vi "Principal Component Regression vs Partial Least Squares Regression.vi"() -> ()   [LabVIEW 2020]
doc: "Created a simple data set with two features. Fitting a PCA estimator to display the two principal components of this data set, i.e., the two directions that explain the most variance in the data."
uses:
  Model/Unsupervised/Decomposition/PCA/Controls/pca_params.ctl
  Model/Unsupervised/Decomposition/PCA/PCA.lvclass
  C:/Users/cipop/TDF Dropbox/2_Technologies de France/1 - Services et Etudes/PLAIY/2 - DEV/PLAIYLAB/code/Model/Model.lvclass
  Model/Unsupervised/Decomposition/PCA/PCA.vi
panel:
  in  "error in":errorcluster
  in  "X":dbl[][](array[numeric])=[[-3.1230621555120366, -3.267402245779568], [-2.7759583555493745, -0.9291009956420317], [-2.5824162791620315, -4.072344785760595], [-1.4924533321482034, -1.9203606695549433], [-0.04152867510525987, 0.38116552193039455], [-0.9895929568838566, 0.35548272004878073], [-1.321002512421451, -1.4319109557167145], [-0.9062030407418514, -0.7201426317829231], [-2.363965378211708, -3.00551409310223], [-0.07622116200586487, -0.9848213835175939], [3.8827997801273813, 5.2682947183614415], [-1.0455682933772348, -2.0118262855175173], [-3.000793770679625, -5.066072884305923], [0.021076191053119836, -0.1712349292866861], [-3.293213004454131, -2.348044580088958], [-0.45156251453811036, -0.13684672563754458], [2.4911990537849347, 0.8654600606814207], [0.49437031989305863, 0.7473930976389208], [-2.6551906571871515, -1.8746011462978966], [0.7965278046955226, 0.6235436957786513], [2.4672057894742827, 1.4246706773928945], [1.8127458791245286, 4.183723187879213], [1.0689101490798731, 0.8028309544259182], [1.6693409342820642, 2.7851759352048475], [2.7779867409191974, 3.056413113478895], [1.28044097132362, 1.9168718091876966], [1.454516472193804, 0.4800380543766737], [-0.17474077869416443, 0.2424933474987974], [-0.2662603373981937, 0.002593279598261611], [1.2360847889518942, 1.079101339057454], [1.2974868876792334, 1.1549241930603973], [2.236292462300943, 0.8312098407203671], [-0.08570535170975882, -0.5221219961580871], [2.4558730848103254, 3.383922938130942], [1.473082668462659, 1.793339539503028], [-1.2719644066222633, -1.366366853019776], [-1.2455615883649316, -2.764076488877849], [-0.31128133394330143, -1.084938213482685], [1.7386890479593449, 1.4459865694538756], [0.4860291194557282, 0.6325831741811381], [1.4607162202673052, 2.668123312217531], [0.023997601243387456, -1.581210861785806], [-3.4400020907207445, -2.0744427796423204], [-1.8557584770801652, -2.3791586256349135], [1.2252785308669916, 2.5511532590490686], [0.03485131421930365, 1.3219094827980622], [-0.8489718087252514, 0.021057633347454585], [-0.954242520882054, -0.3861611991001935], [-0.9401672768593397, 0.7612455190095062], [-0.41752715405613133, -0.07170568835595528], [-2.4167558580489956, -4.2649463448703555], [1.5994216853420016, 2.903701384378012], [0.935056942906058, 3.140150593548995], [1.0700158249093736, 0.4799948638084063], [-3.943985606858868, -3.1045675966732573], [-3.555582951142261, -3.2479521887428753], [0.436774411909285, 2.516790560089131], [0.028405354509702996, 0.8742736180556507], [-1.4858766331534665, -1.9164243034844521], [-1.4917113621038822, -0.7947003467271441], [-0.054206900478580566, -1.2158431671974066], [-1.178420764227316, -0.0014102617409005314], [1.2255635582681221, 1.2899555529512825], [-0.23618032716024984, 1.658692026165808], [-1.3219687145720118, -1.133629585524625], [0.9941620940232232, 1.7385461989049822], [1.0983431465659563, 1.329899833217794], [0.7016338957803231, 1.5369575037307723], [-0.8455726116795177, -1.2164018547360114], [-0.08985373180301681, -1.251281106760939], [2.2382660497620366, 3.102539909775831], [-0.6036790814168229, -0.04728997705352106], [-4.427797625785037, -4.237298506790273], [0.9318628713293798, 2.27033725141622], [2.4139407399635457, 2.365954334709854], [-0.7725163598260496, 0.8831626619431198], [1.6582548882395716, 1.0916356936402005], [0.5055970555135226, -0.09829604362883215], [-1.304497377056593, -2.671363413465319], [2.123201941989344, 2.0476470765576895], [-0.1737072849012109, 1.8165369702193837], [-1.6148002860594206, -1.8144794467292016], [1.5895553483051157, 2.7610553746046356], [2.4517586006380316, 1.2757306514269526], [-2.127795936579116, -2.1797146955158735], [-1.687037561069112, -1.657546670957851], [-1.0800891896009337, -1.95708907640884], [1.357587098949138, 2.3166917679275847], [1.684487467372001, 1.2660220463726513], [0.744043644169997, 0.8966271774157081], [1.295689925648856, 0.0889593754981145], [2.212908959730294, 0.28276797927442476], [-0.20579022578061912, -1.921420302525838], [1.798785393093465, 2.178048879910527], [0.4253096343310593, 2.118694225099275], [1.9993280061041725, 2.6399196575033486], [0.6685277864008033, -0.4346535641530578], [-0.776425902433697, -1.0962709897646585], [-1.7014334411694816, -1.1456806529369103], [-4.266831862548306, -3.6365313912391892], [0.7340165938152251, 0.6156773915555652], [-2.156524327626228, -1.8591647387793435], [-0.22272426785381416, -1.9570194715144735], [0.42157644704371794, -0.2755886336250671], [-0.412047724827981, -0.5892392529116066], [-1.6686018074550817, -1.637365447685474], [-1.0589271731939833, -1.7386939359527704], [1.7732203834350928, 1.6636029951994373], [-0.16778048582484578, 0.19918313987653768], [-3.713200926998545, -4.4275600057892115], [1.7591241647054534, 1.714087615107567], [0.5176111003363346, 1.1154727511926705], [2.5145201228572627, 3.034571758319521], [-0.37870731488022336, -0.20379042066372643], [1.110409630266099, 1.0615214579176058], [2.609136057527492, 2.5631252879627286], [0.6824611972822181, 1.2415185537957432], [1.5077068204105204, 2.59825790632907], [-1.4010279076116303, -3.8226036325343458], [-1.0544580831604022, -0.5355421839959715], [1.259077266138524, 1.0700649156531268], [0.37355186176683475, 0.1289644719074876], [1.3768906865528834, -0.1306023050172932], [-2.462876330674744, -1.7761999881369224], [2.1023768285563813, 0.9453840523307628], [-0.5638865499045511, -1.2689050210099266], [-0.06966776486358095, -0.41680386605849484], [-1.502231764160231, -1.045428970358411], [1.9143630858651652, 0.8104645184180699], [2.301476515109009, 3.356302996730963], [2.2272802260543494, 2.0982191939319432], [1.0129753127016978, 1.1407019415196935], [3.1034650485695434, 3.861303032071852], [-0.9117744561650152, -0.9836728847040506], [0.463620329133252, 0.6493326540176726], [0.7729816660272796, -1.9924010730560782], [-3.4350402393224906, -3.646224067737516], [1.2805629784436563, 1.102047845501593], [-0.7562481528851783, -1.0143643627180428], [2.2902989516589423, 4.866598705110763], [-0.34440836486571075, 0.6622855101700247], [0.35019181744509975, 2.023066391831823], [-0.7879831666210565, -0.29229068871313707], [1.102155845873062, 2.5699813382136005], [-1.8130912584448788, -0.7763241349282213], [1.2868996412809248, 1.0151567928103926], [-3.2610412289082293, -4.960120115268076], [-0.3627145013656148, 0.7629632300366], [-0.4627849749446247, 0.06446751141708973], [0.4691415755908187, 0.9415146073433274], [1.3031172548670646, 3.2755197421109115], [0.5468129888226406, -0.06713894944707846], [-0.8635821125135921, -1.5021255953649117], [2.9016510378335933, 2.014313751071669], [-1.0644734160420157, -1.4237555499359422], [-0.3358678897271853, 0.7326850594809373], [2.240403391217416, 1.8791685691338935], [0.5875201531303886, 0.7923974655491977], [0.21795943160435005, -0.04328232332688953], [0.15732693404684453, 0.07329332353105325], [1.6097290944355735, 1.048439962492894], [0.006536589845641649, -0.9257051563936818], [2.074682549867369, 2.1218886778081125], [-0.9054603158856454, 1.2955334831430163], [0.6775848894798995, 1.7881265800876855], [-0.6208732812742819, -1.9785867891528066], [-0.6665796080587857, -2.027235361483064], [4.082778804652155, 5.454806295039896], [2.6697866153395244, 3.6240263333178833], [0.27325472064938794, 2.0612956521081696], [-1.5321575468236415, -2.2836685408424118], [1.7644644634471083, 0.8108784741798338], [0.8737903876842514, 0.7377434932758122], [0.5219295476248138, 0.7802974932957978], [-1.1370742912796614, -0.9759344513891441], [2.0062115379467023, 0.8618636827982649], [-1.8995543846428702, -2.964692117125013], [1.3476694183914666, 1.0448147458438994], [3.2939016371559027, 3.387541996156069], [0.4723993359108689, 1.2076047997409527], [-1.15662143970013, -1.3613950313055445], [-1.716179145733433, -1.669696577670932], [-0.05723075688290312, 0.10104753431650992], [0.5192135789425586, 0.19922298559988247], [1.0254855678930572, 0.02871548705687116], [0.04955493009300638, -0.9820086854769112], [-1.2624628154709912, -1.751647832684781], [-0.33700311796421617, 0.11957927435606289], [-0.25192758744399957, -1.9429496323234021], [-0.11276460560748963, 0.7890587860400128], [2.6071499866693078, 3.4833953040787584], [4.257203373914415, 3.954168641112636], [0.7922075925398219, -0.8005885735062946], [2.3897611827611946, 1.2789610808487466], [-2.8095189142448405, -3.1444626915200535], [-0.8227685231847532, -1.2045447824707207], [1.4195621605189146, -0.017860496326389086], [0.8759428355501255, 0.23619224516754922], [-2.0079386658467873, -1.1747473904713763], [-2.865050676141875, -2.4888510666693113], [1.5662955642224357, 0.6798126138498647], [-1.451535919349128, -1.3401888755973128], [2.7400188171811104, 3.606925876978513], [-1.376993484663037, -1.5637493342400972], [0.7232607799336566, 0.007598693396809408], [1.9778409324743031, 3.173243734894971], [0.6316594322042454, 0.5010434202148424], [-3.2181946114229407, -3.081792175376673], [-0.6864464432967216, -0.6614831723449329], [-3.4013792813625985, -2.213561355763916], [-1.8374875875250434, -1.5590783880981642], [3.3988179387222597, 4.141794841306994], [0.16654151049915855, 0.29503147353814235], [-0.14335429990191018, -3.0396133959544915], [0.8017062074067494, 1.2291641515886955], [1.5039328123750066, 0.29082534424293593], [-1.5796173846581025, -1.5745941219067074], [1.442732420989098, 2.032925902941954], [-1.3609610156158853, -1.6010154518183417], [-1.3639140932992975, -1.5280525761180117], [1.2524880357581751, 0.263775174168296], [0.04166216316219769, 0.25274334155968015], [-1.3884268772571104, -1.7595823133499298], [-0.25774689097973547, -1.3148944148621475], [1.3508653136453304, 1.4789869785616112], [1.319642108393654, 2.4171677862715444], [-0.9098526917261823, -0.7816334494516979], [-1.6045976678183593, 0.22330509901165885], [1.91266109902782, -0.04865305233923711], [-0.3033301385811629, -0.41108709899179996], [1.3613388751841846, 0.5814760612414922], [0.632355175149752, 0.936460484967083], [-0.41533709348972814, 2.037264740613474], [1.9977090040313212, 1.5272587977725598], [3.6535437912370616, 4.5763467787299845], [3.612227162303425, 3.6988987613221695], [0.8224681920434698, 0.22730150377680097], [-3.3884945786544756, -2.958146009832311], [-1.7247957159551681, -2.96057279232882], [-2.122062605534064, -1.985345376811369], [-1.8072097919734924, -1.0547854685641302], [1.7216027059795702, 1.5877217080760038], [-0.05379126994125172, -2.845819232819154], [-2.7876170627020302, -2.711149183584468], [-0.038385718854680465, 0.1857154274986857], [1.883490221475557, 1.8567462235195495], [-2.489688174081815, -1.5790267308510786], [-4.41913520359936, -5.294065876287195], [1.3544232356882078, 1.060074551262173], [1.7232325775049468, 1.9526385876044559], [-0.615030305926815, -0.7618949409584685], [-1.6914289859234148, -2.2420553953822284], [0.8747548071075235, 0.4236121756401645], [3.5091420955780626, 2.4998362030706187], [1.27687209844225, 2.8708172038884943], [-2.190505332938247, -1.1452401661616056], [3.2196240049641918, 1.7380893892952531], [1.0003390332616595, 1.3650680508415156], [-1.3659393450364132, -0.5144656038865167], [-1.3704498241145897, 0.20805110086691792], [0.8398198656834015, 0.03473116745726451], [3.2387065698138966, 2.8917800427617566], [0.058962729271365366, -0.8615186312394935], [-2.278389544426113, -1.2098377112514116], [3.470865465231734, 5.0024962258386205], [3.4949949933122344, 4.546358154349681], [-2.058440133756621, -2.361956666208289], [2.4180605806504833, 2.241062225498926], [0.5267170334118553, 0.4308287856899863], [0.3922037650228464, 0.3478556487629465], [0.2715833857303947, -0.9456422148243377], [-0.38442623363554035, 1.1368986505003955], [0.8652291962581795, 0.5563569598142126], [-0.4600485979263118, -3.224354540600303], [-1.626505068926789, -2.5820772426607976], [-0.3207747770394916, -0.27774500504463906], [-1.4197924698318296, -1.9563707196356495], [0.45026329081991656, 1.8912850277911297], [3.897889263120339, 4.622608344846892], [2.6218847009640864, 2.2971224664694376], [-3.301918503358635, -3.9445072182586447], [0.5980983822673835, -1.1605311515703456], [1.1036727988509758, 1.5087773664099555], [-0.9052394846508768, -0.4222806869356237], [-0.286581152326219, 0.21385028561419794], [0.19529611899377375, -1.6864994254797279], [-0.45797349218007305, 0.26392005357943715], [-0.787159479405164, -1.3104294108592958], [1.9097056113668347, 1.08266442595462], [-0.3688384402389152, 0.7517408306763018], [3.5676609796297547, 3.520106901625024], [1.4786852325384499, 2.567937854862507], [1.1595631764060415, 0.8757262854092012], [0.12850885753191696, 0.6183429331979667], [2.222714982741702, -0.567649868791737], [-1.1250561201613922, -0.8680941797234533], [0.9230918926925015, -0.0460834151304334], [-0.7775161318321409, -0.5204978618967042], [0.8890384675958839, 0.8224028249598483], [1.6299947777113484, 1.737034604623724], [2.347493068162403, 3.208352087278317], [1.4381732475048934, 1.9471698344513608], [2.6292039709584474, 2.485461468307296], [1.0407882049782182, -0.5113238220891487], [0.005556324020851849, -0.3906779705754937], [3.5538439803439412, 2.829750673293757], [-1.4631289312303253, -0.7888821295209305], [0.008916586803490834, 0.4345989941153663], [-0.5403782600839842, -0.29254559504645045], [-1.347250555438185, -3.1692744353522677], [-0.920914319924806, -1.4873378096284238], [0.5269204220638951, 0.3053384009313589], [1.2537940139225603, 0.19535523435154833], [-1.1665147265552531, 0.37364057244978105], [0.093513478034955, 0.1089378355044669], [1.1969289497510778, 1.2898479034071806], [-0.579340808299716, -1.0717958934999747], [0.5418401684343338, 1.0621254821343125], [1.3871518540368202, 1.9020213022562555], [-2.058859870450213, -1.0055698351979978], [-0.5572580743889034, 0.7750252777585079], [-1.1952913305741795, -2.454736836780727], [2.1710504585102037, 2.2433254470564026], [-1.663659229548592, -2.0396197532244917], [0.1909057669573675, 1.8516586246375306], [0.7248117751784309, -1.5757000392352194], [-0.7930419116869436, -0.39130242838598306], [-0.6053496502382718, -0.24342308533023335], [0.7924702194679163, -0.4458178435735871], [1.1014650790503557, 0.3095040631620988], [2.194647815974929, 1.2673645533636786], [-0.7986299734995203, -0.8401842278411138], [1.076427371070743, 0.590361557660835], [-0.5189273666607129, 0.5181107389127977], [3.1185796730324777, 4.07621747192674], [1.8759760425434933, 0.24001455309733133], [3.6882511189370213, 3.397501359029687], [-0.5659945661531601, -0.25631790868304416], [1.0267792356953098, 2.2776161120246243], [-2.5571117584952785, -2.6035850375003315], [0.39667434295859705, 1.6463244699401323], [-1.697015884505475, -1.0944679858184305], [2.549943341126908, 0.04031386270894255], [-2.6670434695231284, -4.836073937242132], [-1.1710663178312846, 1.11193514414797], [-1.0370037312040556, -0.2296060927953698], [3.4022965339009397, 2.153795558553288], [0.31703103016938305, 1.5170328453298123], [0.9830220952827111, 0.327869632499599], [-0.8863408433744439, 0.08726491256154939], [3.0142623118065925, 2.2899184077158266], [0.7381793918875201, 2.0182559883710582], [-1.4899443101991492, 0.47505983723272427], [-1.5299753764147221, -1.8428449734064318], [-2.200683281973791, -2.3762318136249405], [0.8139974959776535, 1.6733088060051153], [1.3012070802366906, 1.2317712838972], [-2.142724138511322, -2.6355147457163417], [1.5676706177818713, 1.3640815108455078], [-1.4036870284752592, -2.235899804917811], [0.9032482095254041, 0.5316095549219733], [-0.1048680306461782, -0.5276743395776265], [3.10654868304228, 2.7376487264274454], [0.8996072234342821, 2.3645898520792086], [-1.6469468287653113, -1.3288775619629154], [1.2569886232341434, 0.6291117224774245], [1.3825518183614636, 0.5299815733661939], [-2.96809283759535, -5.856163832139279], [-0.26864177990074245, -1.6629602867747066], [0.6830262509118721, -0.2288548356945198], [2.5359995778633646, 1.7990511683375452], [-2.8325829835562106, -3.483085507802404], [0.9786502802942577, 1.7375619196610135], [-0.38917068681952627, 0.29498654297282095], [2.85893758833089, 3.692951756604405], [-0.4188069240043504, -2.235259449979505], [-1.6174100262715765, -0.1321807925773849], [-0.399880858182534, 0.3885523335432996], [-0.7429834365204397, -1.6183238913486533], [0.7439682635667801, -0.763532170258383], [0.6087952002408533, 0.9970227959380888], [-1.208130482541127, -1.4003638298165517], [-0.6203578782535882, -1.8878346580051244], [0.15816134674915444, 0.2069024291874486], [-2.947034847793407, -3.7032427149738663], [0.8139297881848236, 0.9831818085265928], [1.4198554423873546, 1.8780334410347004], [1.5291293914860344, -0.07171646728053027], [0.2609372440839284, -0.02466723538576078], [2.733373856654159, 3.156302477625673], [-2.731540342492316, -2.678299704704095], [-0.31843500922551893, -1.7814005142598568], [-0.8651051790044021, -0.8656901968249724], [-1.0929890818562262, -0.8474377869987186], [2.2693504341962245, 2.6355022937487944], [1.2787741081500954, 1.4570685771900003], [0.8053721918997865, 2.3257993574464724], [1.8845413134480253, 1.2827950401595642], [0.4332625159514308, -0.6170390604743649], [1.1309091358313803, 0.46543061444201195], [-2.7389631000635877, -2.409942390996509], [0.29715997261618543, -0.059096738697375806], [-1.7648830538641134, -1.6588379084976252], [-0.8098342542303217, -0.983419174848098], [2.8490564365119493, 3.245366539535865], [0.5469818218218501, 1.3215217597268143], [-1.3327725099693453, -2.262627605526309], [-1.671300338166604, -0.15420475267771994], [0.23475126973647575, 2.0392821314088647], [1.3976109084014514, 1.6738795459248283], [0.012483862154438138, 0.02678422660621726], [1.6903103499824905, 1.375955554167373], [0.9349088036598671, 1.4461850785080053], [-1.69581354756115, 0.3303051102285527], [-2.0030365858565453, -2.8986736768884596], [-1.0523053584168611, -0.19751356363005357], [-0.014604477604199681, -0.09020424069506962], [-0.5334084054496566, 0.27898756733552466], [1.5707059786005015, 1.5129488266880518], [-0.9386423534646182, -0.7817236922291085], [-0.20498604410723562, -0.6294225827406893], [-2.710402267345278, -0.9638458247090663], [-0.5720567592413217, -0.8776836771066427], [-0.9707872460297131, -1.710831000537503], [1.2224172382367764, 1.4773892473173524], [4.866096797993505, 4.535228435590456], [1.274575964535802, 0.08662637606688761], [1.9328212640493883, 1.8240330604736266], [2.9259401227779573, 3.0285107103579816], [0.8717684583975712, 1.0557054728884336], [-1.9972076922404132, -2.1768898968189525], [-0.08621011832696712, 0.0024318747254457942], [0.1494567185870651, -0.8888203077939019], [0.030203522245500214, 0.35913606891712635], [1.8188012239641353, 3.053976764156676], [-1.4614558927868648, -2.386690272734532], [0.8527592988684873, 0.08655910710867148], [-0.6078363182205679, -1.8293807536026017], [0.811621530337562, 0.058187442126031996], [0.8428916910973735, -0.8848330794344621], [-1.6944362280376684, -3.0108434593527527], [0.01080008027026938, -0.20991361900119385], [1.7186504264175788, 1.0986619822674097], [-1.2764189334839497, -2.057481351539185], [-0.03413646202226567, -0.8800336742492111], [0.8258818879552619, 1.4696993146199153], [-1.4475385682874315, -1.8924428744785824], [1.318285055438903, 3.6494634674968003], [2.212608182012837, 0.9967586412006207], [-4.080266944389543, -5.239902630110594], [2.7696543808710223, 2.553420163102244], [-0.7059558377868579, -0.6339614543665482], [0.4662067449671522, 2.460025786797859], [1.47442371312839, 0.49928991920495225], [-2.2749594004920333, -1.2930260534996312], [2.0755754155352033, 0.9819279562653516], [-0.6455873074521481, -2.9070932973531423], [1.5279157532984535, 2.817247840914131], [0.22789128866510036, -0.007513360265690758], [-0.5043253200072187, -0.7553994913345637], [1.4875747403346902, 3.092981009262771], [-2.296583079320573, -2.495896288503137], [-1.2835636161340298, 0.9360540972134122], [0.5911229085958843, 0.42583559426313494], [-1.3628247442155224, -0.06724078893033747], [-2.499519454801301, -3.2214931249143404], [0.20236804862574487, -1.204945440637395], [0.9499529452317834, 0.2410005434958568], [0.7955531531932145, 2.7009250740907147], [1.5844851970506961, 1.3134528201083575], [-1.2754349685037303, -0.1458549700435694], [-2.221203634228492, 0.26896313700335817], [-0.010246627064372793, 0.25896426727783955], [-1.197146425416905, 0.09033274699517913], [-0.7784963784255408, -1.040759273947651], [1.4400551168008056, 1.9560341158886414], [-2.1046146142836855, -2.9143756867832957], [-1.0016285377222187, -0.9244911528502744], [-1.011711759983442, -2.0374348651075103], [-3.218443553718094, -5.1394361237513655], [0.11958198355079591, 1.1240114722471453], [-0.9194291980603966, -0.21576432765500997], [0.858798512210938, 0.9354036666818466], [-0.8311016590782153, 0.6630476094565352], [-1.5530636170732999, -0.9986481714029916], [0.5870193562785356, 1.7080619078056454], [-1.0907362662863045, 0.1678515378858968], [-3.171082437828916, -4.064739124222517], [1.118166817712333, 0.4146824162878398], [0.434765429650407, 0.11297119898313987], [-0.5196225204010211, -0.7648580329869736], [0.047686708105601605, 1.171669601458295], [1.326682609855824, 2.019868187198832], [0.29679198010765656, 1.1092798817006027], [-2.1334624920697975, -2.8360273424808455], [-0.8214924599742897, -0.7824161218224821], [1.1971646972046448, 1.6654812144533282], [-0.691309034270523, -0.38349374226264993], [0.2793166078051734, 0.42840848964944067], [2.08225088820075, 2.0828147820518317]]
  out "error out":errorcluster caption="sortie d'erreur"
  out "explained_variance_":dbl[](array[numeric])
  out "components_":dbl[][](array[numeric])
  out "XY Graph":cluster{"X":dbl[], "Y":dbl[]}[](graph) caption="2-dimensional dataset with principal components"
  in  "R/W params":T1={"n_components"={"n_components_type"="int", "n_components_int"=2, "n_components_float"=0.0}, "copy"=TRUE, "whiten"=FALSE, "svd_solver"="auto", "tol"=0.0, "iterated_power"={"iterated_power_type"="auto", "iterated_power_int"=0.0}, "random_state"=0.0}
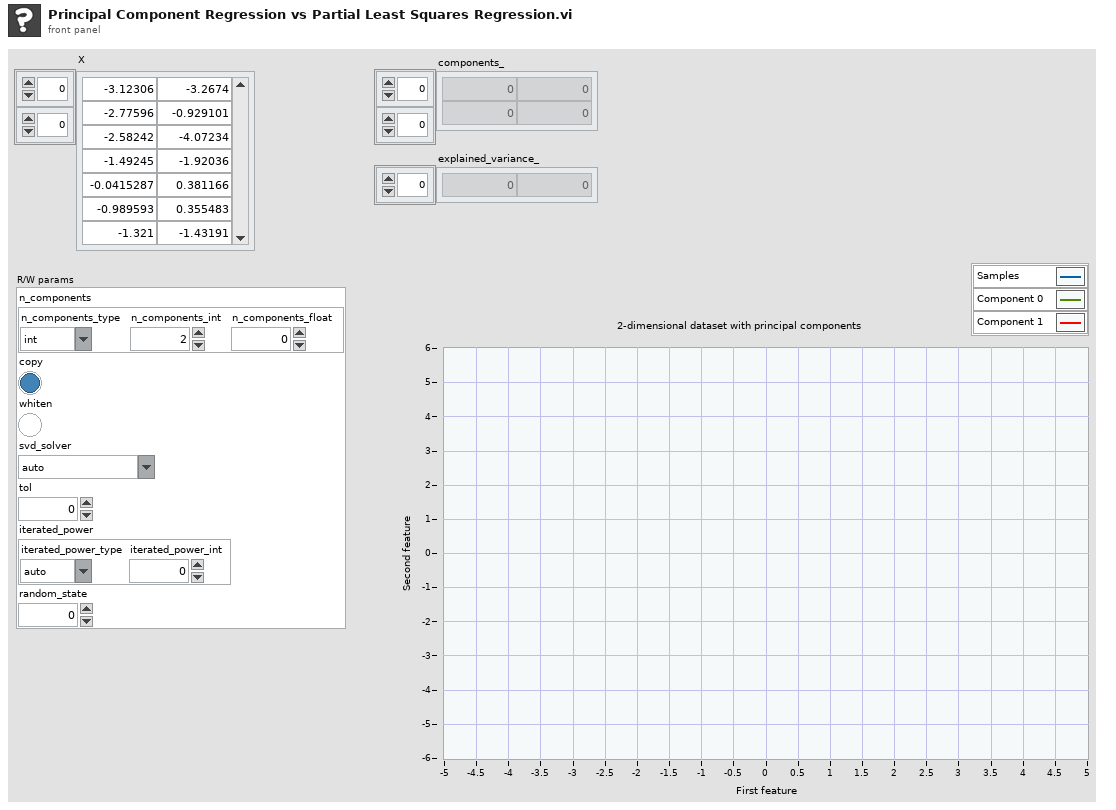
[diagram p1: front panel]
types:
  T1 = typedef "pca_params.ctl" = cluster{"n_components":cluster{"n_components_type":string, "n_components_int":i32, "n_components_float":dbl}, "copy":bool, "whiten":bool, "svd_solver":string, "tol":dbl, "iterated_power":cluster{"iterated_power_type":string, "iterated_power_int":dbl}, "random_state":dbl}
  T2 = typedef "pca_attributes.ctl" = cluster{"components_":dbl[][], "explained_variance_":dbl[], "explained_variance_ratio_":dbl[], "singular_values_":dbl[], "mean_":dbl[], "n_components_":dbl, "n_features_":dbl, "n_samples_":dbl, "noise_variance_":dbl}
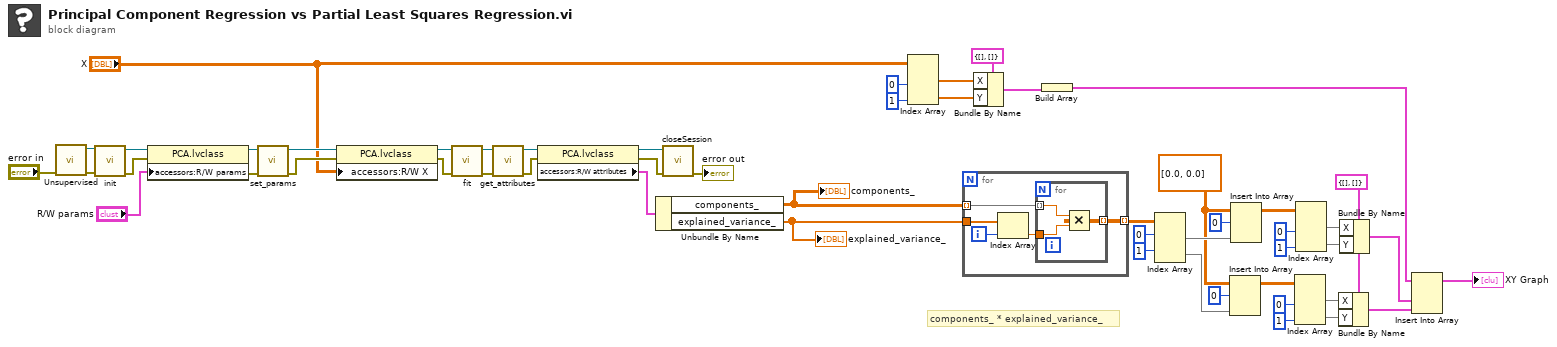
[diagram p0: block diagram]
diagram:
  w7 = dbl[][] [[0.0, 0.0]]
  w9 = cluster{"X":dbl[], "Y":dbl[]} {"X"=[], "Y"=[]}
  # "components_ * explained_variance_"
  n1 = call-poly "Unsupervised.vi"("error in"="error in") -> ("error out"=w43:errorcluster, "out"=w44:refnum<class "PCA.lvclass">)  [unwired: 9 in]
  n2 = call-dynamic "init.vi"("error in (no error)"=w43, "Model en entrée"=w44) -> ("error out"=w47:errorcluster, "Model en sortie"=w51:refnum<class "PCA.lvclass">)  [unwired: 8 in]
  n3 = property class="PCA.lvclass"(reference=w51, error in=w47, "accessors:R/W params"="R/W params") -> (reference out=w50:refnum<class "PCA.lvclass">, error out=w52:errorcluster)
  n4 = call-dynamic "set_params.vi"("error in (no error)"=w52, "PCA.lvclass 2"=w50) -> ("error out"=w48:errorcluster, "PCA.lvclass"=w49:refnum<class "PCA.lvclass">)  [unwired: 8 in]
  n5 = property class="PCA.lvclass"(reference=w49, error in=w48, "accessors:R/W X"="X") -> (reference out=w41:refnum<class "PCA.lvclass">, error out=w40:errorcluster)
  n6 = call-dynamic "fit.vi"("error in (no error)"=w40, "Decomposition.lvclass 2"=w41) -> ("error out"=w4:errorcluster, "Decomposition.lvclass"=w5:refnum<class "PCA.lvclass">)  [unwired: 8 in]
  n7 = call-dynamic "get_attributes.vi"("error in (no error)"=w4, "PCA.lvclass 2"=w5) -> ("error out"=w38:errorcluster, "PCA.lvclass"=w39:refnum<class "PCA.lvclass">)  [unwired: 8 in]
  n8 = property class="PCA.lvclass"(reference=w39, error in=w38) -> (reference out=w46:refnum<class "PCA.lvclass">, error out=w45:errorcluster, "accessors:R/W attributes"=w32:T2)
  n9 = Unbundle By Name(w32) -> ("components_"=w30:dbl[][], "explained_variance_"=w31:dbl[])
  "components_" <- w30
  "explained_variance_" <- w31
  n10 = call-dynamic "closeSession.vi"("error in"=w45, "Python en entrée"=w46) -> ("error out"=→"error out":errorcluster)  [unwired: 8 in, 1 out]
  n11 = Index Array(array="X", index (col) #1=0 ("disabled index (col)"), index (col) #2=1 ("index (col)")) -> (element #1=w34:dbl[], element #2=w33:dbl[])  [unwired: 2 in]
  n12 = for {
    tunnel: w30 -> [w56] mode=indexing
    tunnel: w31 -> [w55]
    tunnel: [w57] -> w29 mode=indexing
    i -> [w54]
    n13 = Index Array(array=w55, index=w54) -> (element=w53:dbl)
    n14 = for {
      tunnel: [w60] -> w57 mode=indexing
      tunnel: w56 -> [w59] mode=indexing
      tunnel: w53 -> [w58]
      n15 = Multiply(x=w59, y=w58) -> (x*y=w60:dbl)
    }
  }
  n16 = Bundle By Name(cluster=cluster{"X":dbl[], "Y":dbl[]} {"X"=[], "Y"=[]}, "X"=w34, "Y"=w33) -> (w20:cluster{"X":dbl[], "Y":dbl[]})
  n17 = Build Array(w20) -> (w19:cluster{"X":dbl[], "Y":dbl[]}[])
  n18 = Index Array(array=w29, index (row) #1=0 ("index (row)"), index (row) #2=1 ("index (row)")) -> (element #1=w25:dbl[], element #2=w8:dbl[])  [unwired: 2 in]
  n19 = Insert Into Array(array=w7, index (row)=0 ("index"), new element=w8) -> (w11:dbl[][])  [unwired: 1 in]
  n20 = Insert Into Array(array=w7, index (row)=0 ("index"), new element=w25) -> (w26:dbl[][])  [unwired: 1 in]
  n21 = Index Array(array=w11, index (col) #1=0 ("disabled index (col)"), index (col) #2=1 ("index (col)")) -> (element #1=w14:dbl[], element #2=w15:dbl[])  [unwired: 2 in]
  n22 = Index Array(array=w26, index (col) #1=0 ("disabled index (col)"), index (col) #2=1 ("index (col)")) -> (element #1=w22:dbl[], element #2=w21:dbl[])  [unwired: 2 in]
  n23 = Bundle By Name(cluster=w9, "X"=w14, "Y"=w15) -> (w6:cluster{"X":dbl[], "Y":dbl[]})
  n24 = Bundle By Name(cluster=w9, "X"=w22, "Y"=w21) -> (w18:cluster{"X":dbl[], "Y":dbl[]})
  n25 = Insert Into Array(array=w19, new element #1=w18, new element #2=w6) -> (→"XY Graph":cluster{"X":dbl[], "Y":dbl[]}[])  [unwired: 1 in]
